vi "SetAxisRelativeMove.vi"(8 "error in (no error)":errorcluster, 10 "RelativeMovement":i32, 11 "Picomoto8742ControllerClass in":refnum<class "Picomoto8742ControllerClass.lvclass">) -> (0 "error out":errorcluster, 3 "Picomoto8742ControllerClass out":refnum<class "Picomoto8742ControllerClass.lvclass">)   [LabVIEW 2020, in "Picomoto8742ControllerClass.lvclass"]
doc: "Send a relative move requsest relative to the active axis, to the physical device"
uses:
  Picomoto8742ControllerClass.lvclass
  Picomoto8742ControllerClass.lvclass/Picomoto8742ControllerClass.ctl
  Picomotor8742Axis.lvclass
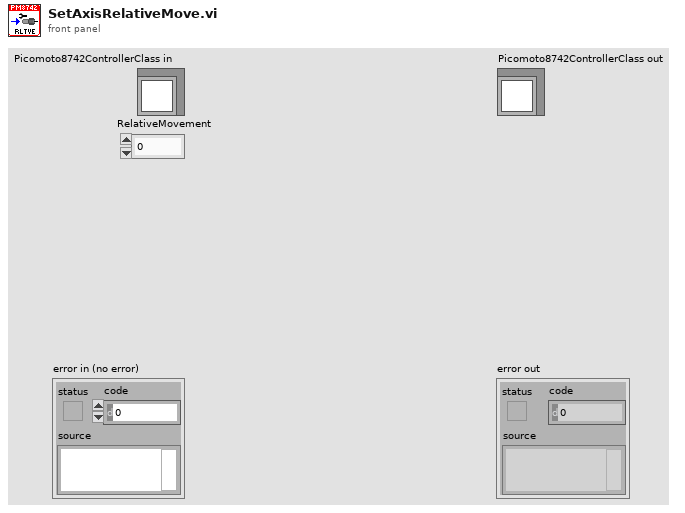
[diagram p1: front panel]
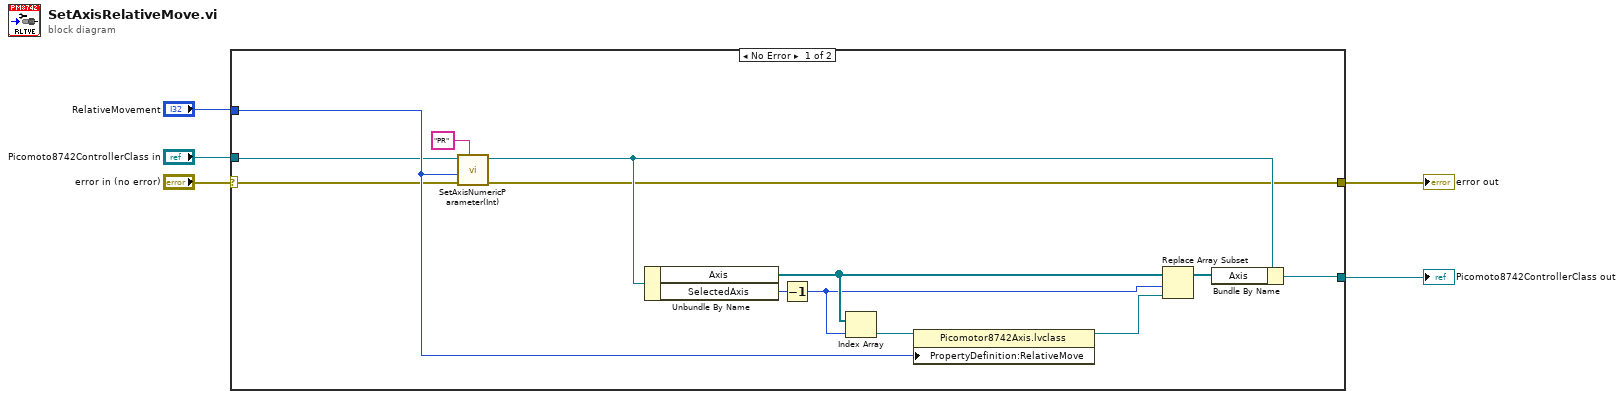
[diagram p0: block diagram]
diagram:
  n1 = case shown="No Error" "error in (no error)" {
    selector: "error in (no error)" -> [w8 w20]
    tunnel: [w6 w20] -> w4
    tunnel: [w16 w19] -> w2
    tunnel: "Picomoto8742ControllerClass in" -> [w9 w19]
    tunnel: "RelativeMovement" -> [w10 _]
    frame No Error {
      n2 = call "SetAxisNumericParameter(Int).vi"("CMD"="PR" ("string"), "error in (no error)"=w8, "ParameterValue"=w10, "Picomoto8742ControllerClass in"=w9) -> ("error out"=w6:errorcluster, "Picomoto8742ControllerClass Out"=w7:refnum<class "Picomoto8742ControllerClass.lvclass">)  [unwired: 6 in]
      n3 = Unbundle By Name(w7) -> ("Axis"=w14:refnum<class "Picomotor8742Axis.lvclass">[], "SelectedAxis"=w13:u32)
      n4 = Decrement(x=w13) -> (x-1=w11:u32)
      n5 = Index Array(array=w14, index=w11) -> (element=w12:refnum<class "Picomotor8742Axis.lvclass">)
      n6 = property class="Picomotor8742Axis.lvclass"(reference=w12, "PropertyDefinition:RelativeMove"=w10) -> (reference out=w18:refnum<class "Picomotor8742Axis.lvclass">)  [unwired: 1 in, 1 out]
      n7 = Replace Array Subset(array=w14, new element=w18, index=w11) -> (w17:refnum<class "Picomotor8742Axis.lvclass">[])
      n8 = Bundle By Name(cluster=w7, "Axis"=w17) -> (w16:refnum<class "Picomoto8742ControllerClass.lvclass">)
    }
    frame Error {
    }
  }
  "error out" <- w4
  "Picomoto8742ControllerClass out" <- w2
